vi "Read_Configure_INI.vi"(8 "error in (no error)":errorcluster) -> (0 "error out":errorcluster)   [LabVIEW 2011]
uses:
  Global.vi
  <vilib>/Utility/config.llb/Read Key (String).vi
  <vilib>/Utility/config.llb/Read Key (U32).vi
  <vilib>/Utility/config.llb/NI_LVConfig.lvlib
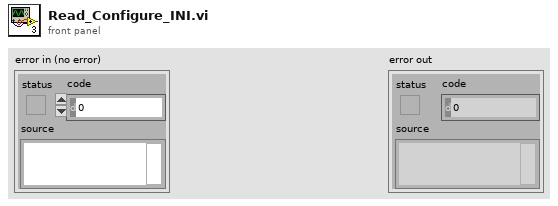
[diagram p1: front panel]
types:
  T1 = typedef "NI_LVConfig.lvlib/Config Data RefNum.ctl" = refnum<k1>
  T2 = cluster{"Label1":string, "Label2":string, "Model_Name":string, "Test_Time":string, "Test_Result":string, "DSN":string, "Table_Name":string}
  T3 = cluster{"Label1":string, "Label2":string, "Test_Time":string, "Model_Name":string, "Test_Result":string}
  T4 = cluster{"Fix_SN1":string, "Offset_SN1":u32, "Fix_SN1_Length":u32}
  T5 = cluster{"Fix_SN2":string, "Offset_SN2":u32, "Fix_SN2_Length":u32}
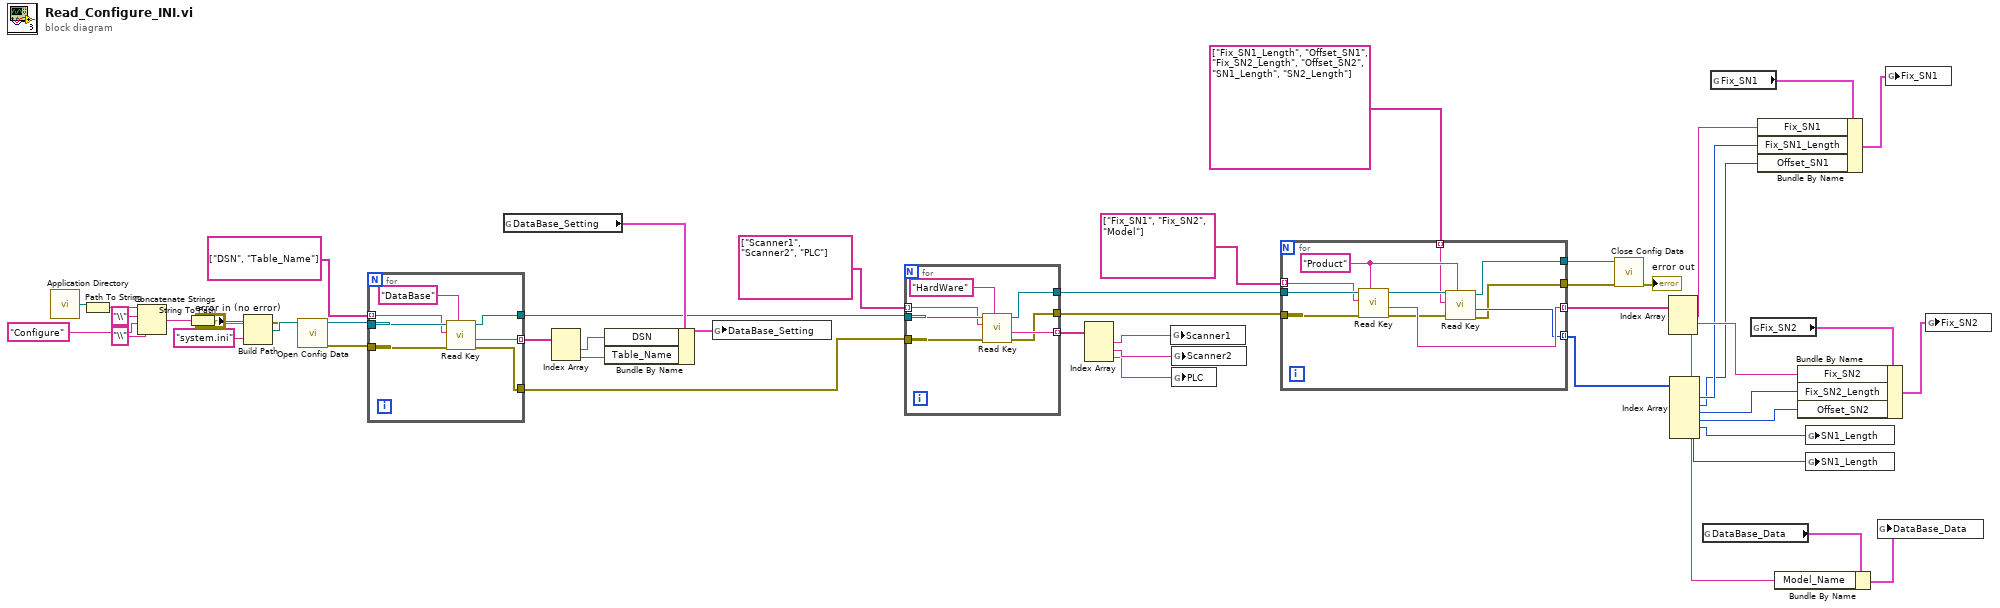
[diagram p0: block diagram]
diagram:
  n1 = call <vilib>:"Application Directory.vi"() -> ("Application Directory"=w49:path)
  n2 = Path To String(path=w49) -> (string=w48:string)
  n3 = Concatenate Strings(w48, "\\" ("string"), "Configure" ("string"), "\\" ("string")) -> (w44:string)
  n4 = String To Path(string=w44) -> (path=w43:path)
  n5 = Build Path(base path=w43, name or relative path="system.ini") -> (appended path=w41:path)
  n6 = call <vilib>:"Open Config Data.vi"("error in (no error)"="error in (no error)", "configuration file path"=w41) -> ("error out"=w39:errorcluster, "refnum"=w40:T1)  [unwired: 7 in, 1 out]
  n7 = for {
    tunnel: w40 -> [w56]
    tunnel: w39 -> [w55]
    tunnel: string[] ["DSN", "Table_Name"] -> [w53] mode=indexing
    tunnel: [w52] -> w35 mode=indexing
    tunnel: [w51] -> w32
    tunnel: [w50] -> w31
    n8 = call-poly <vilib>:"Read Key.vi"("section"="DataBase", "error in (no error)"=w55, "key"=w53, "refnum"=w56) -> ("error out"=w50:errorcluster, "value"=w52:string, "refnum out"=w51:T1)  [unwired: 4 in, 1 out]
  }
  n9 = global read "Global.vi" "DataBase_Setting"() -> (w37:T2)
  n10 = Index Array(array=w35) -> (element #1=w34:string, element #2=w33:string)  [unwired: 2 in]
  n11 = Bundle By Name(cluster=w37, "DSN"=w34, "Table_Name"=w33) -> (w36:T2)
  n12 = global write "Global.vi" "DataBase_Setting"(w36) -> ()
  n13 = for {
    tunnel: w32 -> [w63]
    tunnel: w31 -> [w62]
    tunnel: string[] ["Scanner1", "Scanner2", "PLC"] -> [w60] mode=indexing
    tunnel: [w59] -> w29 mode=indexing
    tunnel: [w58] -> w24
    tunnel: [w57] -> w23
    n14 = call-poly <vilib>:"Read Key.vi"("section"="HardWare", "error in (no error)"=w62, "key"=w60, "refnum"=w63) -> ("error out"=w57:errorcluster, "value"=w59:string, "refnum out"=w58:T1)  [unwired: 4 in, 1 out]
  }
  n15 = Index Array(array=w29) -> (element #1=w28:string, element #2=w27:string, element #3=w26:string)  [unwired: 3 in]
  n16 = global write "Global.vi" "Scanner1"(w28) -> ()
  n17 = global write "Global.vi" "Scanner2"(w27) -> ()
  n18 = global write "Global.vi" "PLC"(w26) -> ()
  n19 = for {
    tunnel: w24 -> [w74]
    tunnel: w23 -> [w73]
    tunnel: string[] ["Fix_SN1", "Fix_SN2", "Model"] -> [w72] mode=indexing
    tunnel: [w71] -> w25 mode=indexing
    tunnel: string[] ["Fix_SN1_Length", "Offset_SN1", "Fix_SN2_Length", "Offset_SN2", "SN1_Length", "SN2_Length"] -> [w68] mode=indexing
    tunnel: [w67] -> w11 mode=indexing
    tunnel: [w66] -> w4
    tunnel: [w64] -> w3
    w69 = "Product" ("section")
    n20 = call-poly <vilib>:"Read Key.vi"("section"=w69, "error in (no error)"=w73, "key"=w72, "refnum"=w74) -> ("error out"=w65:errorcluster, "value"=w71:string, "refnum out"=w70:T1)  [unwired: 4 in, 1 out]
    n21 = call-poly <vilib>:"Read Key.vi"("section"=w69, "error in (no error)"=w65, "key"=w68, "refnum"=w70) -> ("error out"=w64:errorcluster, "value"=w67:u32, "refnum out"=w66:T1)  [unwired: 4 in, 1 out]
  }
  n22 = call <vilib>:"Close Config Data.vi"("error in (no error)"=w3, "refnum"=w4) -> ("error out"=→"error out":errorcluster)  [unwired: 8 in, 1 out]
  n23 = Index Array(array=w25) -> (element #1=w19:string, element #2=w16:string, element #3=w13:string)  [unwired: 3 in]
  n24 = Index Array(array=w11) -> (element #1=w10:u32, element #2=w9:u32, element #3=w8:u32, element #4=w7:u32, element #5=w6:u32, element #6=w5:u32)  [unwired: 6 in]
  n25 = global read "Global.vi" "DataBase_Data"() -> (w15:T3)
  n26 = global read "Global.vi" "Fix_SN1"() -> (w21:T4)
  n27 = global read "Global.vi" "Fix_SN2"() -> (w17:T5)
  n28 = Bundle By Name(cluster=w21, "Fix_SN1"=w19, "Fix_SN1_Length"=w10, "Offset_SN1"=w9) -> (w20:T4)
  n29 = Bundle By Name(cluster=w15, "Model_Name"=w13) -> (w14:T3)
  n30 = Bundle By Name(cluster=w17, "Fix_SN2"=w16, "Fix_SN2_Length"=w8, "Offset_SN2"=w7) -> (w18:T5)
  n31 = global write "Global.vi" "SN1_Length"(w6) -> ()
  n32 = global write "Global.vi" "SN1_Length"(w5) -> ()
  n33 = global write "Global.vi" "DataBase_Data"(w14) -> ()
  n34 = global write "Global.vi" "Fix_SN1"(w20) -> ()
  n35 = global write "Global.vi" "Fix_SN2"(w18) -> ()
